vi "setSpeedTarget_ShootDualTalonSRX.vi"(7 "Right Speed Target\nFt/SEC":dbl format="%.4f", 10 "Left Speed Target\nFT/SEC":dbl format="%.4f") -> ()   [LabVIEW 2019, in "ShootDualTalonSRX_Motor_Pair.lvlib"]
uses:
  ShootDualTalonSRX_Motor_Pair.lvlib
  globals_ShootDualTalonSRX.vi
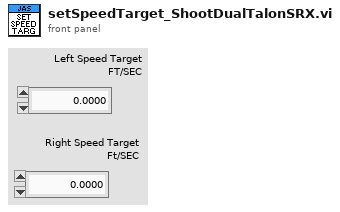
[diagram p1: front panel]
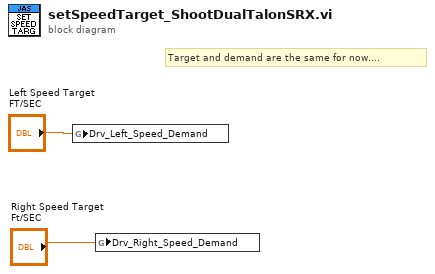
[diagram p0: block diagram]
diagram:
  # "Target and demand are the same for now...."
  n1 = global write "globals_ShootDualTalonSRX.vi" "Drv_Left_Speed_Demand"("Left Speed Target\nFT/SEC") -> ()
  n2 = global write "globals_ShootDualTalonSRX.vi" "Drv_Right_Speed_Demand"("Right Speed Target\nFt/SEC") -> ()
